vi "Decide Action.vi"(8 "error in (no error)":errorcluster, 11 "MyMouse in":refnum<class "MyMouse.lvclass">) -> (0 "error out":errorcluster, 2 "Action":T1, 3 "MyMouse out":refnum<class "MyMouse.lvclass">)   [LabVIEW 2020, in "Mouse.lvlib" / "MyMouse.lvclass"]
uses:
  MyMouse.lvclass
  C:/dev/lv/2020/SoL/sol-maze/ProjectTemplates/Source/SummerOfLabVIEW/Summer of LabVIEW - Maze/template/Maze/Mouse/Mouse.lvclass
  Maze/Action.ctl
  Maze/Mouse/Mouse.lvclass
  Maze/Maze.lvlib
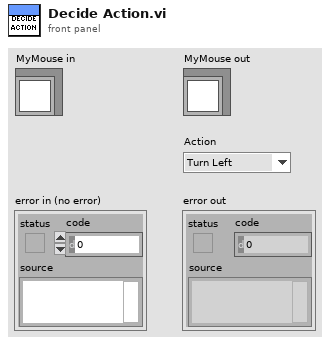
[diagram p1: front panel]
types:
  T1 = typedef "Maze.lvlib/Action.ctl" = enum16{"Turn Left", "Turn Right", "Forward", "*Drop Marker", "*Pickup Marker"}
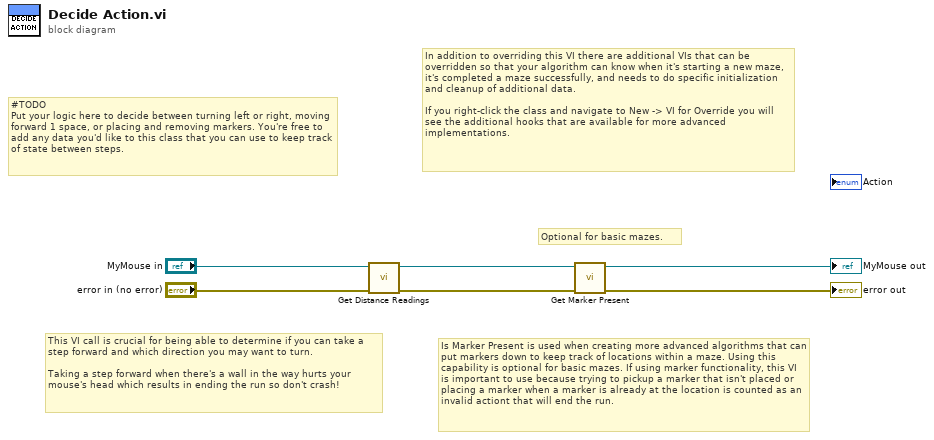
[diagram p0: block diagram]
diagram:
  # "Optional for basic mazes."
  # "Is Marker Present is used when creating more advanced algorithms that can put markers down to keep track of locations within a maze. Using this capability is optional for basic mazes. If using marker functionality, this VI is important to use because trying to pickup a marker that isn't placed or placing a marker when a marker is already at the location is counted as an invalid actiont that will end the run."
  # "In addition to overriding this VI there are additional VIs that can be overridden so that your algorithm can know when it's starting a new maze, it's completed a maze successfully, and needs to do specific initialization and cleanup of additional data.\n\nIf you right-click the class and navigate to New -> VI for Override you will see the additional hooks that are available for more advanced implementations."
  # "This VI call is crucial for being able to determine if you can take a step forward and which direction you may want to turn.\n\nTaking a step forward when there's a wall in the way hurts your mouse's head which results in ending the run so don't crash!"
  # "#TODO\nPut your logic here to decide between turning left or right, moving forward 1 space, or placing and removing markers. You're free to add any data you'd like to this class that you can use to keep track of state between steps."
  n1 = call "Get Distance Readings.vi"("error in (no error)"="error in (no error)", "Mouse in"="MyMouse in") -> ("error out"=w3:errorcluster, "Mouse out"=w4:refnum<class "MyMouse.lvclass">)  [unwired: 7 in, 1 out]
  n2 = call "Get Marker Present.vi"("error in (no error)"=w3, "Mouse in"=w4) -> ("error out"=→"error out":errorcluster, "Mouse out"=→"MyMouse out":refnum<class "MyMouse.lvclass">)  [unwired: 7 in, 1 out]
